vi "plates.vi"() -> ()   [LabVIEW 2016]
uses:
  C:/Users/UsphereLab/Documents/GitHub/Optlev/LabView Code/Tilt Stage/CmdLib.dll
  Tilt Stage/CmdLib.dll
panel:
  in  "stop":bool
  in  "on/off":bool
  in  "Z steps":dbl
  in  "Y steps":dbl
  in  "tilt stage config 2":T1
  in  "Y error in (no error)":errorcluster
  in  "Run thetaY?":bool
  in  "Run thetaZ?":bool
  in  "Z error in (no error)":errorcluster
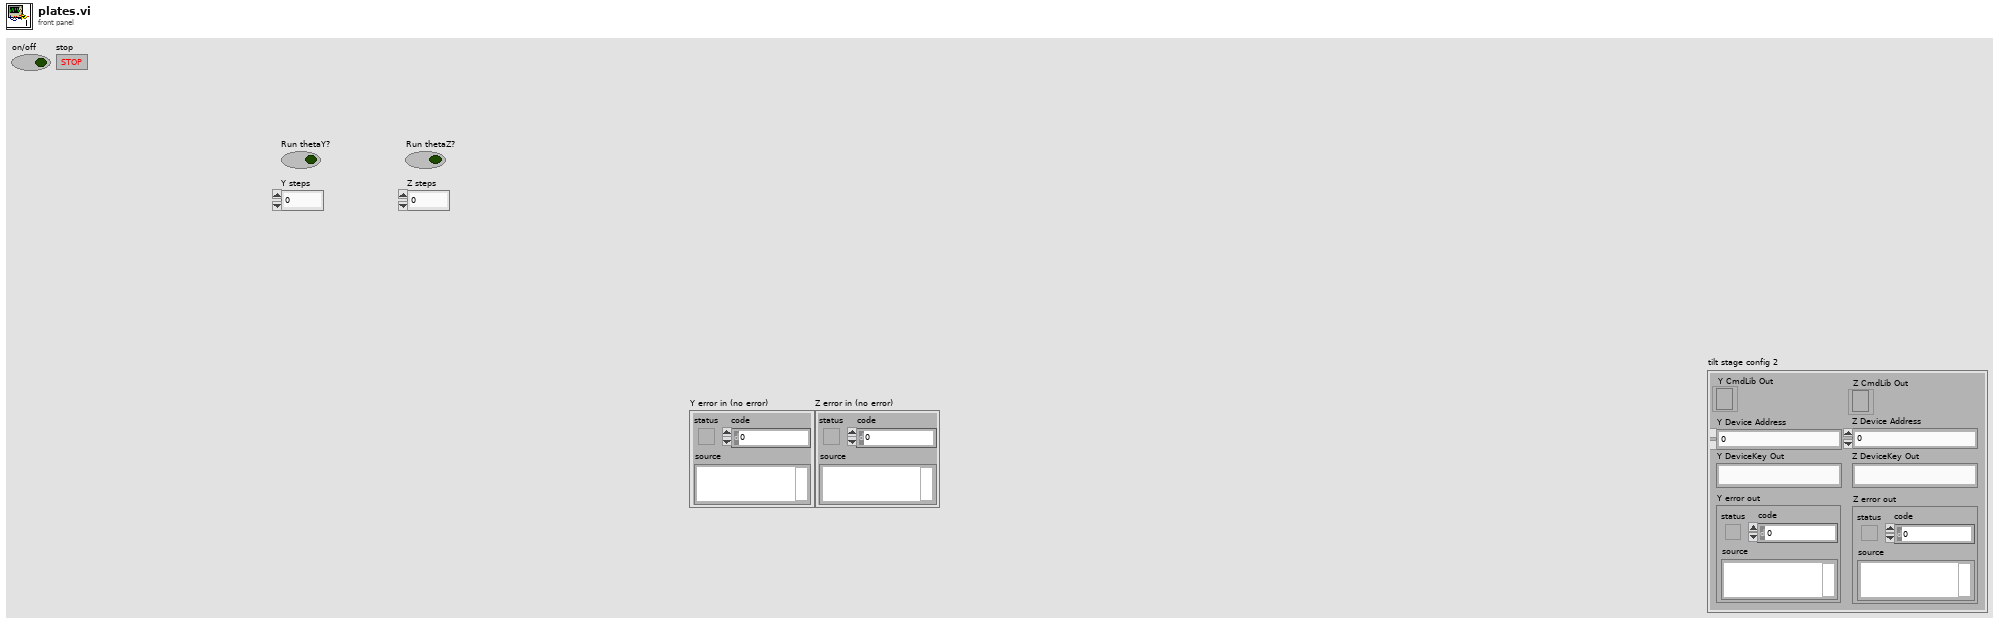
[diagram p1: front panel]
types:
  T1 = cluster{"Y error out":errorcluster, "Y CmdLib Out":refnum<k24>, "Y Device Address":i32, "Y DeviceKey Out":string, "Z error out":errorcluster, "Z CmdLib Out":refnum<k24>, "Z Device Address":i32, "Z DeviceKey Out":string}
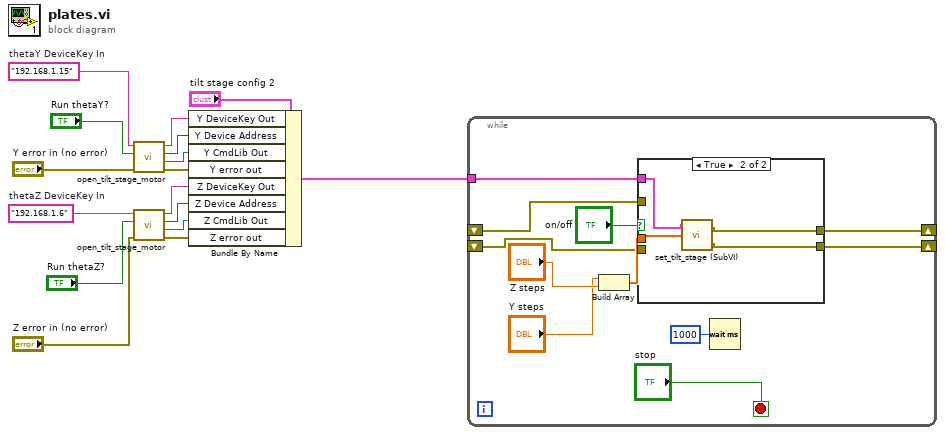
[diagram p0: block diagram]
diagram:
  w11 = "192.168.1.15"  # thetaY DeviceKey In
  w12 = "192.168.1.6"  # thetaZ DeviceKey In
  n1 = call "open_tilt_stage_motor.vi"("error in (no error)"="Y error in (no error)", "Open device?"="Run thetaY?", "DeviceKey In"=w11) -> ("error out"=w5:errorcluster, "CmdLib Out"=w4:refnum<k24>, "Device Address"=w3:i32, "DeviceKey Out"=w2:string)  [unwired: 1 in]
  n2 = call "open_tilt_stage_motor.vi"("error in (no error)"="Z error in (no error)", "Open device?"="Run thetaZ?", "DeviceKey In"=w12) -> ("error out"=w9:errorcluster, "CmdLib Out"=w8:refnum<k24>, "Device Address"=w7:i32, "DeviceKey Out"=w6:string)  [unwired: 1 in]
  n3 = Bundle By Name(cluster="tilt stage config 2", "Y DeviceKey Out"=w2, "Y Device Address"=w3, "Y CmdLib Out"=w4, "Y error out"=w5, "Z DeviceKey Out"=w6, "Z Device Address"=w7, "Z CmdLib Out"=w8, "Z error out"=w9) -> (w1:T1)
  n4 = while {
    tunnel: w1 -> [w27]
    shift-right: [w20] -> _
    shift-left: _ -> [w18]
    shift-right: [w19] -> _
    shift-left: _ -> [w17]
    stop <- "stop" stop-if-true
    n5 = Build Array("Y steps", "Z steps") -> (w24:dbl[])
    n6 = case shown="True" "on/off" {
      tunnel: w27 -> [_ w31]
      tunnel: w24 -> [_ w30]
      tunnel: [w29 w33] -> w20
      tunnel: [w28 w32] -> w19
      tunnel: w18 -> [w29 _]
      tunnel: w17 -> [w28 _]
      frame False {
      }
      frame True {
        n7 = call "set_tilt_stage (SubVI).vi"("Tot Stage Arr"=w30, "tilt stage config"=w31) -> ("thetaZ error out"=w32:errorcluster, "thetaY error out"=w33:errorcluster)  [unwired: 1 in]
      }
    }
    n8 = Wait (ms)(milliseconds to wait=u32 1000) -> ()  [unwired: 1 out]
  }
